vi "Check for Infinite Values.vi"(7 "Positive?":bool, 11 "Pressure Limit":dbl) -> (3 "element":string)   [LabVIEW 2015]
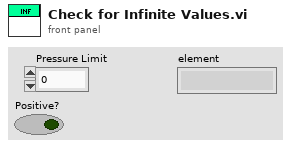
[diagram p1: front panel]
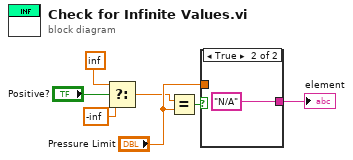
[diagram p0: block diagram]
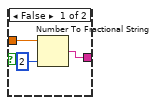
[diagram p2: hidden frame]
diagram:
  n1 = Select(t=inf, s="Positive?", f=-inf) -> (s? t:f=w1:dbl)
  n2 = Equal?(x=w1, y="Pressure Limit") -> (x = y?=w5:bool)
  n3 = case shown="True" w5 {
    tunnel: [w8 "N/A" ("element")] -> w7
    tunnel: "Pressure Limit" -> [w10 _]
    frame False {
      n4 = Number To Fractional String(number=w10, precision (6)=i16 2) -> (F-format string=w8:string)  [unwired: 2 in]
    }
    frame True {
    }
  }
  "element" <- w7
